vi "Unregister Listener.vi"(8 "error in (no error)":errorcluster, 10 "Listener NQR":refnum<class "Message Enqueuer.lvclass">, 11 "Broadcast Registry In":refnum<class "Broadcast Registry.lvclass">) -> (0 "error out":errorcluster, 3 "Broadcast Registry Out":refnum<class "Broadcast Registry.lvclass">)   [LabVIEW 2016, in "Data Broadcasting.lvlib" / "Broadcast Registry.lvclass"]
doc: "Unregisters a Listener from receiving the next broadcast of this Registry's data message. Listeners are referenced by their <b>NQR</b> (Enqueuer).\n\n-------------\nCopyright (c) 2013, Staab Engineering, a Texas Limited Liability Company\nAll rights reserved.\n\nRedistribution and use in source and binary forms, with or without modification, are permitted provided that the following conditions are met:\n\n1. Redistributions of source code must retain the above copyright notice, this list of conditions and the following disclaimer.\n2. Redistributions in binary form must reproduce the above copyright notice, this list of conditions and the following disclaimer in the documentation and/or other materials provided with the distribution.\n\nTHIS SOFTWARE IS PROVIDED BY THE COPYRIGHT HOLDERS AND CONTRIBUTORS \"AS IS\" AND ANY EXPRESS OR IMPLIED WARRANTIES, INCLUDING, BUT NOT LIMITED TO, THE IMPLIED WARRANTIES OF MERCHANTABILITY AND FITNESS FOR A PARTICULAR PURPOSE ARE DISCLAIMED. IN NO EVENT SHALL THE COPYRIGHT HOLDER OR CONTRIBUTORS BE LIABLE FOR ANY DIRECT, INDIRECT, INCIDENTAL, SPECIAL, EXEMPLARY, OR CONSEQUENTIAL DAMAGES (INCLUDING, BUT NOT LIMITED TO, PROCUREMENT OF SUBSTITUTE GOODS OR SERVICES; LOSS OF USE, DATA, OR PROFITS; OR BUSINESS INTERRUPTION) HOWEVER CAUSED AND ON ANY THEORY OF LIABILITY, WHETHER IN CONTRACT, STRICT LIABILITY, OR TORT (INCLUDING NEGLIGENCE OR OTHERWISE) ARISING IN ANY WAY OUT OF THE USE OF THIS SOFTWARE, EVEN IF ADVISED OF THE POSSIBILITY OF SUCH DAMAGE."
uses:
  <userlib>/_Frameworks/Staab/AF Data Broadcasting/Data Broadcasting/Broadcast Registry/Broadcast Registry.lvclass
  <vilib>/ActorFramework/Message Enqueuer/Message Enqueuer.lvclass
  <userlib>/_Frameworks/Staab/AF Data Broadcasting/Data Broadcasting/Broadcast Registry/Broadcast Registry.lvclass/Broadcast Registry.ctl
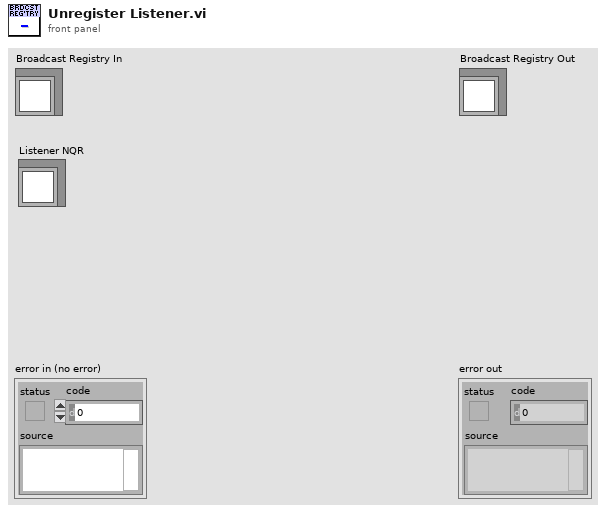
[diagram p1: front panel]
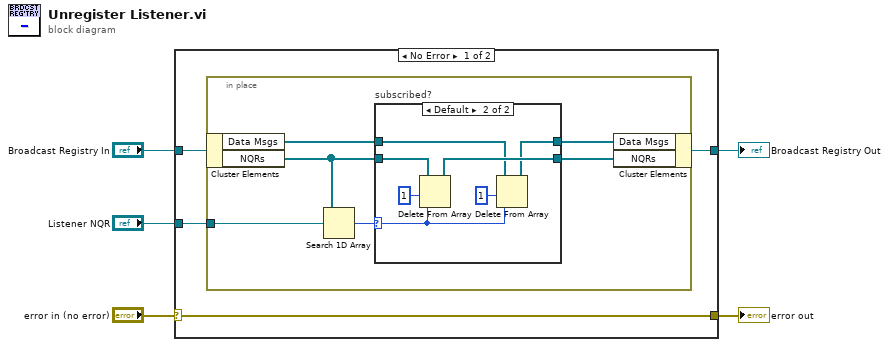
[diagram p0: block diagram]
diagram:
  n1 = case shown="No Error" "error in (no error)" {
    selector: "error in (no error)" -> [w9 w26]
    tunnel: [w9 w26] -> w4
    tunnel: [w6 w25] -> w2
    tunnel: "Broadcast Registry In" -> [w8 w25]
    tunnel: "Listener NQR" -> [w7 _]
    frame No Error {
      n2 = in-place {
        in-place-border: w7 -> [w13]
        n3 = in-place-cluster #1(w8) -> ("Data Msgs"=w10:refnum<class "Data Msg.lvclass">[], "NQRs"=w14:refnum<class "Message Enqueuer.lvclass">[])
        n4 = Search 1D Array(1D array=w14, element=w13) -> (index of element=w12:i32)  [unwired: 1 in]
        n5 = case "subscribed?" shown="Default" w12 {
          selector: w12 -> [_ w18]
          tunnel: w14 -> [w17 w24]
          tunnel: [w17 w22] -> w15
          tunnel: [w16 w19] -> w11
          tunnel: w10 -> [w16 w20]
          frame -1 {
          }
          frame Default {
            n6 = Delete From Array(array=w24, length=1, index=w18) -> (array with subset deleted=w22:refnum<class "Message Enqueuer.lvclass">[])  [unwired: 1 out]
            n7 = Delete From Array(array=w20, length=1, index=w18) -> (array with subset deleted=w19:refnum<class "Data Msg.lvclass">[])  [unwired: 1 out]
          }
        }
        n8 = in-place-cluster #1("Data Msgs"=w11, "NQRs"=w15) -> (w6:refnum<class "Broadcast Registry.lvclass">)
      }
    }
    frame Error {
    }
  }
  "error out" <- w4
  "Broadcast Registry Out" <- w2
